vi "BoolCmd_Send_OnEdge.vi"(7 "Command Name":string, 11 "Value":bool) -> (0 "error out":errorcluster)   [LabVIEW 2019, in "Trajectory_Library.lvlib"]
uses:
  Trajectory_Library.lvlib
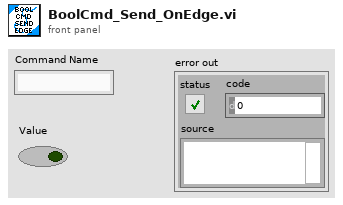
[diagram p1: front panel]
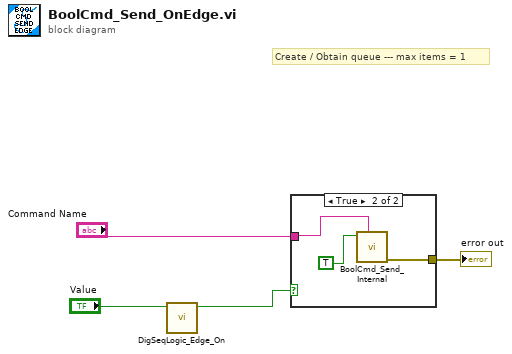
[diagram p0: block diagram]
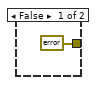
[diagram p2: hidden frame]
diagram:
  # "Create / Obtain queue --- max items = 1"
  n1 = call "DigSeqLogic_Edge_On.vi"("Input"="Value") -> ("On Edge"=w3:bool)  [unwired: 10 in]
  n2 = case shown="True" w3 {
    tunnel: "Command Name" -> [_ w7]
    tunnel: [errorcluster {"status"=FALSE, "code"=0, "source"=""} ("error out") w8] -> w1
    frame False {
    }
    frame True {
      n3 = call "BoolCmd_Send_Internal.vi"("Command Name"=w7, "Value"=TRUE) -> ("error out"=w8:errorcluster)  [unwired: 9 in]
    }
  }
  "error out" <- w1
